vi "getSavePath.vi"(0 "beam_name":string, 5 "Polarizer":string, 7 "Analyzer":string(combo), 9 "prefix":string, 11 "suffix":string) -> (4 "appended filename":string)   [LabVIEW 2023]
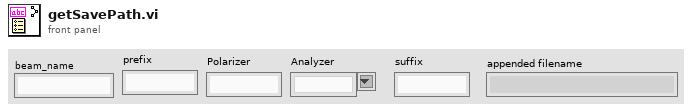
[diagram p1: front panel]
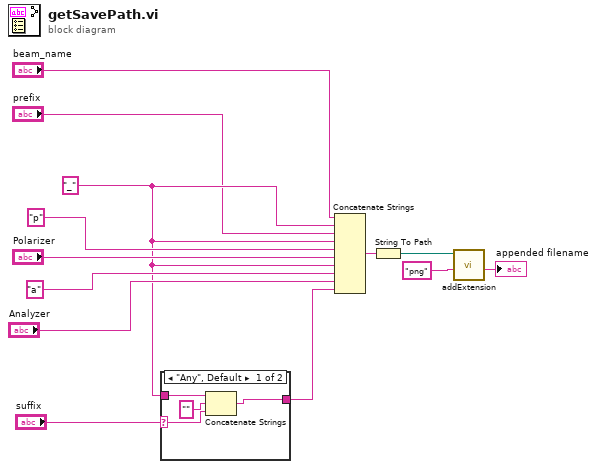
[diagram p0: block diagram]
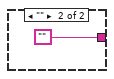
[diagram p2: hidden frame]
diagram:
  w2 = "_" ("string")
  n1 = case shown="\"Any\", Default" "suffix" {
    selector: "suffix" -> [w15 _]
    tunnel: w2 -> [w17 _]
    tunnel: [w14 ""] -> w12
    frame "Any", Default {
      n2 = Concatenate Strings(w17, "" ("string"), w15) -> (w14:string)
    }
    frame "" {
    }
  }
  n3 = Concatenate Strings("beam_name", w2, "prefix", w2, "p" ("string"), "Polarizer", w2, "a" ("string"), "Analyzer", w12) -> (w7:string)
  n4 = String To Path(string=w7) -> (path=w8:path)
  n5 = call "addExtension.vi"("Extension"="png" ("pattern label"), "In path"=w8) -> ("Out path"=→"appended filename":string)  [unwired: 8 in, 1 out]
